vi "Monitor TestState.vi"(8 "error in (no error)":errorcluster, 10 "Address (0)":i32, 11 "VISA resource name":refnum<visa-resource-name>) -> (0 "error out":errorcluster, 1 "measured humidity":dbl, 2 "measured temp":dbl, 3 "VISA resource name out":refnum<visa-resource-name>, 4 "number of alarms":i32, 5 "Mode":T1)   [LabVIEW 2021, in "Environment Chamber.lvlib" / "Climatic Chamber.lvlib"]
doc: "<b>Test area state monitor</B>\n\nReturns the chamber test area state."
uses:
  Climatic Chamber.lvlib
  Private/Type Defs/Mode Enum.ctl
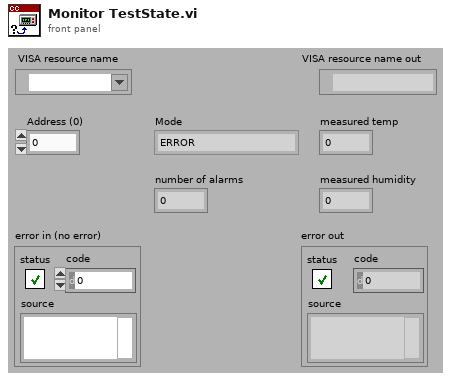
[diagram p1: front panel]
types:
  T1 = typedef "Environment Chamber.lvlib/Climatic Chamber.lvlib/Mode Enum.ctl" = enum16{"ERROR", "OFF", "STANDBY", "CONSTANT", "RUN", "RUN PAUSE", "RUN END HOLD", "RMT RUN", "RMT RUN PAUSE", "RMT RUN END HOLD"}
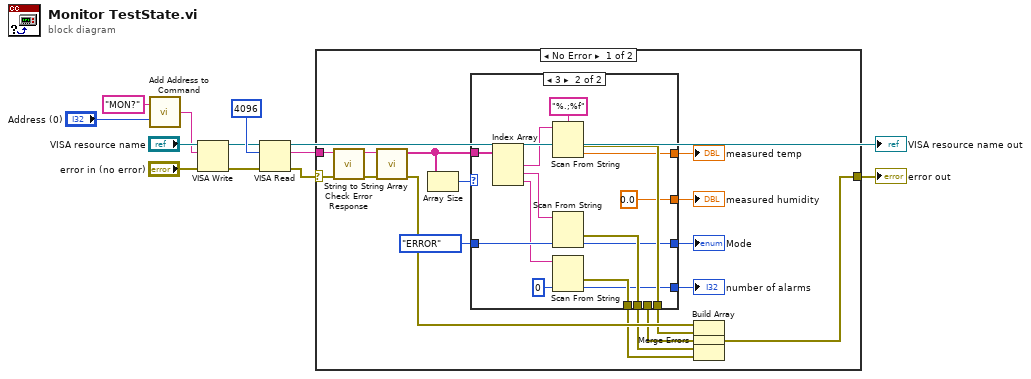
[diagram p0: block diagram]
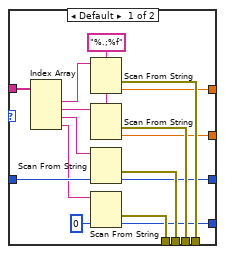
[diagram p2: hidden frame]
diagram:
  n1 = call "Add Address to Command.vi"("Address (0)"="Address (0)", "Command"="MON?") -> ("Command OUT"=w4:string)
  n2 = VISA Write(VISA resource name="VISA resource name", write buffer=w4, error in (no error)="error in (no error)") -> (VISA resource name out=w9:refnum<visa-resource-name>, error out=w8:errorcluster)  [unwired: 1 out]
  n3 = VISA Read(VISA resource name=w9, byte count=u32 4096, error in (no error)=w8) -> (VISA resource name out=→"VISA resource name out":refnum<visa-resource-name>, read buffer=w2:string, error out=w3:errorcluster)  [unwired: 1 out]
  n4 = case shown="No Error" w3 {
    selector: w3 -> [w28 w61]
    tunnel: w2 -> [w30 _]
    tunnel: [w18 w61] -> w1
    frame No Error {
      n5 = call "Check Error Response.vi"("error in (no error)"=w28, "read String"=w30) -> ("error out"=w27:errorcluster, "String out"=w29:string)  [unwired: 7 in, 1 out]
      n6 = call "String to String Array.vi"("error in (no error)"=w27, "String received"=w29) -> ("error out"=w26:errorcluster, "Array Data"=w24:string[])  [unwired: 8 in]
      n7 = Array Size(array=w24) -> (size(s)=w25:i32)
      n8 = case shown="3" w25 {
        tunnel: w24 -> [w42 w57]
        tunnel: [w40 w55] -> w23
        tunnel: [w37 0.0] -> w22
        tunnel: Mode_Enum."ERROR" ("MODE") -> [w35 w53]
        tunnel: [w34 w52] -> w20
        tunnel: [w32 w51] -> w19
        tunnel: [w46 w60] -> w17
        tunnel: [w45 _] -> w16
        tunnel: [w44 w59] -> w15
        tunnel: [w43 w58] -> w14
        frame Default {
          w39 = "%.;%f" ("format string")
          n9 = Index Array(array=w42) -> (element #1=w41:string, element #2=w38:string, element #3=w36:string, element #4=w33:string)  [unwired: 4 in]
          n10 = Scan From String(format string=w39, input string=w41) -> (error out=w46:errorcluster, output 1=w40:dbl)  [unwired: 3 in, 2 out]
          n11 = Scan From String(format string=w39, input string=w38) -> (error out=w45:errorcluster, output 1=w37:dbl)  [unwired: 3 in, 2 out]
          n12 = Scan From String(input string=w36, default 1=w35) -> (error out=w44:errorcluster, output 1=w34:T1)  [unwired: 3 in, 2 out]
          n13 = Scan From String(input string=w33, default 1=0) -> (error out=w43:errorcluster, output 1=w32:i32)  [unwired: 3 in, 2 out]
        }
        frame 3 {
          n14 = Index Array(array=w57) -> (element #1=w56:string, element #2=w49:string, element #3=w48:string)  [unwired: 3 in]
          n15 = Scan From String(format string="%.;%f", input string=w56) -> (error out=w60:errorcluster, output 1=w55:dbl)  [unwired: 3 in, 2 out]
          n16 = Scan From String(input string=w49, default 1=w53) -> (error out=w59:errorcluster, output 1=w52:T1)  [unwired: 3 in, 2 out]
          n17 = Scan From String(input string=w48, default 1=0) -> (error out=w58:errorcluster, output 1=w51:i32)  [unwired: 3 in, 2 out]
        }
      }
      "measured temp" <- w23
      "measured humidity" <- w22
      "Mode" <- w20
      "number of alarms" <- w19
      n18 = Build Array(w26, w17, w16, w15, w14) -> (w13:errorcluster[])
      n19 = Merge Errors(w13) -> (w18:errorcluster)
    }
    frame Error {
    }
  }
  "error out" <- w1
